vi "Set Digital Pin Mode.vi"(8 "Error In":errorcluster, 9 "Pin Mode (Input)":T4, 10 "Digital I/O Pin":u8, 11 "Arduino Resource":T1={"COM Port"="", "Board Type"=enum."ChipKit Uno32", "Connection Type"=enum."USB / Serial", "Baud Rate (115200)"=15, "Bytes Per Packet (15)"=15}) -> (0 "Error Out":errorcluster, 3 "Arduino Resource":T1={"COM Port"="", "Board Type"=enum."ChipKit Uno32", "Connection Type"=enum."USB / Serial", "Baud Rate (115200)"=15, "Bytes Per Packet (15)"=15})   [LabVIEW 2011, in "LabVIEW Interface for ChipKit.lvlib"]
doc: "Configures the specified digital I/O pin (D0 - D13) as either input or output."
uses:
  LabVIEW Interface for ChipKit.lvlib
  Private/Type Defs/Pin Mode.ctl
  Private/Type Defs/Chipkit Resource.ctl
  Private/Type Defs/Board Type.ctl
  Private/Type Defs/Connection Type.ctl
  Private/Type Defs/Command.ctl
  Private/Type Defs/Pin Type.ctl
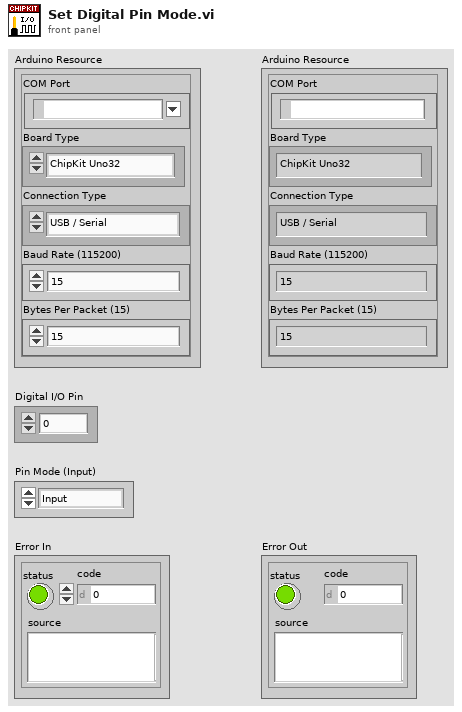
[diagram p1: front panel]
types:
  T1 = typedef "LabVIEW Interface for ChipKit.lvlib/Chipkit Resource.ctl" = cluster{"COM Port":refnum<visa-resource-name>, "Board Type":T2, "Connection Type":T3, "Baud Rate (115200)":u32, "Bytes Per Packet (15)":u32}
  T2 = typedef "LabVIEW Interface for ChipKit.lvlib/Board Type.ctl" = enum16{"ChipKit uC32", "ChipKit Uno32", "ChipKit Max32"}
  T3 = typedef "LabVIEW Interface for ChipKit.lvlib/Connection Type.ctl" = enum8{"USB / Serial", "XBEE", "BlueSmirf (Bluetooth)"}
  T4 = typedef "LabVIEW Interface for ChipKit.lvlib/Pin Mode.ctl" = enum16{"Input", "Output"}
  T5 = typedef "LabVIEW Interface for ChipKit.lvlib/Pin Type.ctl" = enum8{"Analog", "Digital", "PWM", "Tone"}
  T6 = typedef "LabVIEW Interface for ChipKit.lvlib/Command.ctl" = enum8{"setArduinoMode", "flushSerial", "setPinMode", "digitalWritePin", "digitalWritePort", "tone", "digitalReadPin", "digitalReadPort", "analogReadPin", "analogReadPort", "pwmWritePin", "pwmWritePort", "sevenSegment_Configure", "sevenSegment_Write", "I2C Init", "I2C Write", "I2C Read", "SPI Init", "SPI Set Bit Order", "SPI Set Clock Divider", "SPI Set Data Mode", "SPI Send / Receive", "SPI Close", "Servo Set Num Servos", "Servo Config Servo", "Servo Write Angle", "Servo Read Angle", "Servo Write Pulse Width", "Servo Read Pulse Width", "Servo Detach", "LCD Init", "LCD Set Size", "LCD Set Cursor Mode", "LCD Clear", "LCD Set Cursor Position", "LCD Print", "LCD Display Power", "LCD Scroll Display", "LCD Autoscroll", "LCD Print Direction", "LCD Create Custom Char", "LCD Print Custom Char", "contAcqOn", "contAcqOff", "getFirmwareVersion", "FiniteSampleStart", "NA", "NA2", "Configure Stepper", "Stepper Write", "Stepper Detach", "Stepper Steps To Go", "Configure Digital Port"}
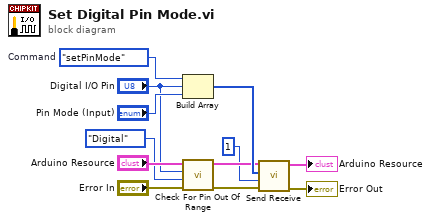
[diagram p0: block diagram]
diagram:
  w12 = Command."setPinMode"  # Command
  n1 = Build Array(w12, "Digital I/O Pin", "Pin Mode (Input)") -> (w7:u16[])
  n2 = call "Check For Pin Out Of Range.vi"("Error In"="Error In", "Pin Type"=Pin_Type."Digital", "User Pin Number"="Digital I/O Pin", "Arduino Resource"="Arduino Resource") -> ("Error Out"=w5:errorcluster, "Arduino Resource"=w6:T1)  [unwired: 6 in]
  n3 = call "Send Receive.vi"("Error In"=w5, "Bytes To Read (0)"=u8 1, "Data"=w7, "ChipKit Resource"=w6) -> ("Error Out"=→"Error Out":errorcluster, "ChipKit Resource"=→"Arduino Resource":T1)  [unwired: 5 in, 1 out]
